vi "Request voltage CH3 (SubVI).vi"() -> (3 "Request voltage CH3 / Z":string)   [LabVIEW 2018]
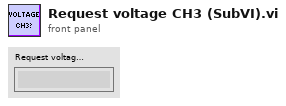
[diagram p1: front panel]
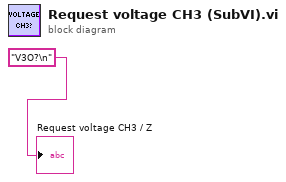
[diagram p0: block diagram]
diagram:
  "Request voltage CH3 / Z" <- "V3O?\n" ("format string")
